vi "Kikusui PLZ-Default Instrument Setup.vi"(8 "error in":errorcluster, 11 "Kikusui PLZ Setting In":T1={"VISA Resource Name"="", "Baud Rate"=19200, "Stop Bits"=20, "Wait For Read(ms)"=0} {"Stop Bits" items=["1.0"=10, "2.0"=20]; "Baud Rate" items=["2400"=2400, "4800"=4800, "9600"=9600, "19200"=19200]}) -> (0 "error out":errorcluster, 3 "Kikusui PLZ Setting Out":T1={"VISA Resource Name"="", "Baud Rate"=19200, "Stop Bits"=20, "Wait For Read(ms)"=0} {"Stop Bits" items=["1.0"=10, "2.0"=20]; "Baud Rate" items=["2400"=2400, "4800"=4800, "9600"=9600, "19200"=19200]})   [LabVIEW 2018]
uses:
  Data Def/Kikusui PLZ-Setting.ctl
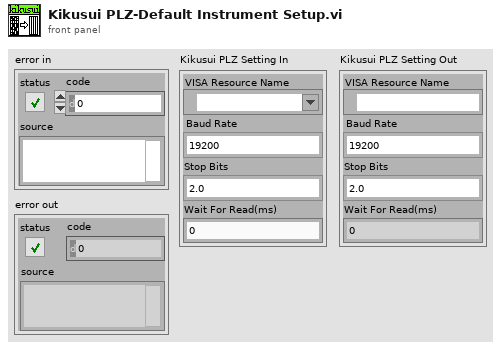
[diagram p1: front panel]
types:
  T1 = typedef "Kikusui PLZ-Setting.ctl" = cluster{"VISA Resource Name":refnum<visa-resource-name>, "Baud Rate":u32, "Stop Bits":u16, "Wait For Read(ms)":u32}
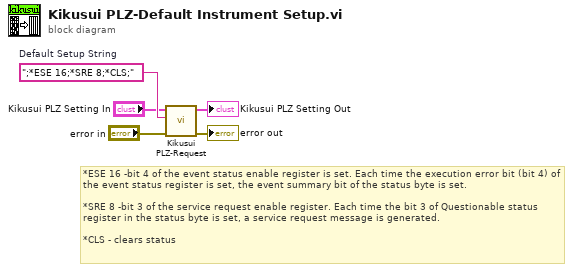
[diagram p0: block diagram]
diagram:
  w5 = ";*ESE 16;*SRE 8;*CLS;"  # Default Setup String
  # "*ESE 16 -bit 4 of the event status enable register is set. Each time the execution error bit (bit 4) of the event status register is set, the event summary bit of the status byte is set.\n\n*SRE 8 -bit 3 of the service request enable register. Each time the bit 3 of Questionable status register in the status byte is set, a service request message is generated. \n\n*CLS - clears status"
  n1 = call "Kikusui PLZ-Request.vi"("error in"="error in", "Command"=w5, "Kikusui PLZ Setting In"="Kikusui PLZ Setting In") -> ("error out"=→"error out":errorcluster, "Kikusui PLZ Setting Out"=→"Kikusui PLZ Setting Out":T1)  [unwired: 6 in, 1 out]
